vi "get child modifications.vi"(8 "error in":errorcluster, 11 "VI modification collection in":refnum<class "VI modification collection.lvclass">) -> (0 "error out":errorcluster, 3 "modifications":refnum<class "VI modification.lvclass">[](array[class]))   [LabVIEW 2013, in "VI modification collection.lvclass"]
uses:
  VI modification collection.lvclass
  VI modification.lvclass
  <vilib>/CEF_TreeControl/Node/NISE_CEF_Node.lvclass/NISE_CEF_Node.ctl
  <vilib>/CEF_TreeControl/Node/ReadChildren.vi
  <vilib>/CEF_TreeControl/Node/NISE_CEF_Node.lvclass
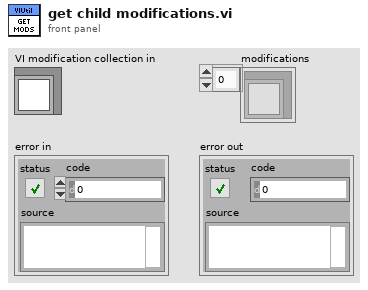
[diagram p1: front panel]
types:
  T1 = typedef "NISE_CEF_Node.lvclass/NodeRef.ctl" = refnum<data-value>
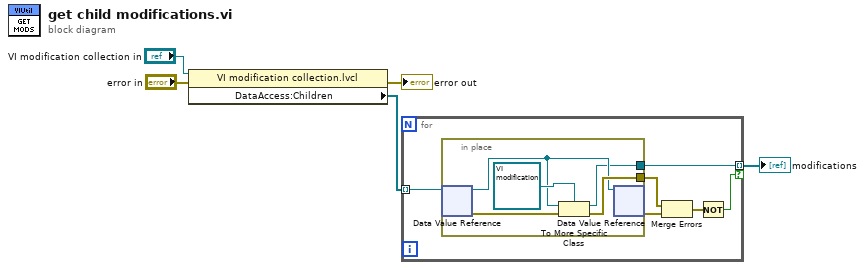
[diagram p0: block diagram]
diagram:
  n1 = property class="VI modification collection.lvcl"(reference="VI modification collection in", error in="error in") -> (error out=→"error out":errorcluster, "DataAccess:Children"=w4:T1[])  [unwired: 1 out]
  n2 = for {
    tunnel: w4 -> [w9] mode=indexing
    tunnel: [w8] -> w5 mode=indexing if=w6
    n3 = in-place {
      in-place-border: [w15] -> w11
      in-place-border: [w12] -> w8
      n4 = in-place-dvr #1(w9) -> (w13:refnum<class "NISE_CEF_Node.lvclass">, w16:errorcluster)
      n5 = To More Specific Class(target class=refnum<class "VI modification.lvclass"> refnum ("VI modification"), reference=w13, error in=w16) -> (specific class reference=w12:refnum<class "VI modification.lvclass">, error out=w15:errorcluster)
      n6 = in-place-dvr #1(w13) -> (w10:errorcluster)  [unwired: 1 out]
    }
    n7 = Merge Errors(w11, w10) -> (w7:errorcluster)
    n8 = Not(x=w7) -> (.not. x?=w6:bool)
  }
  "modifications" <- w5
